vi "PCU_Get_Device_ID.vi"(8 "error in (no error)":errorcluster, 11 ".NET Reference in":refnum<k24>) -> (0 "error out":errorcluster, 2 "id":string[](array[string]), 3 "Reference out":refnum<k24>)   [LabVIEW 2017]
uses:
  D:/test/FULLband-sts/Fullband_Sample/DLL/InstrumentDLL.dll
  DLL/InstrumentDLL.dll
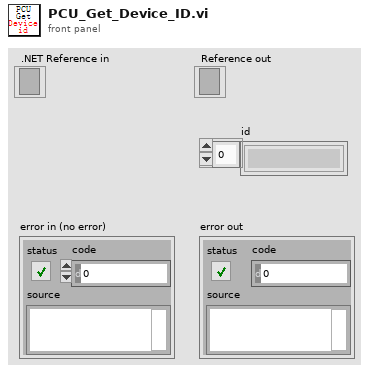
[diagram p1: front panel]
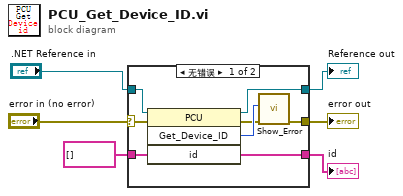
[diagram p0: block diagram]
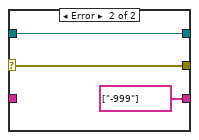
[diagram p2: hidden frame]
diagram:
  n1 = case shown="无错误" "error in (no error)" {
    selector: "error in (no error)" -> [w7 w17]
    tunnel: [w14 string[] ["-999"] ("id")] -> w6
    tunnel: string[] [] ("id") -> [w13 _]
    tunnel: ".NET Reference in" -> [w12 w16]
    tunnel: [w11 w16] -> w3
    tunnel: [w8 w17] -> w2
    frame No Error {
      n2 = invoke on="调用节点" class="PCU" method="Get_Device_ID"(reference=w12, error in=w7, "id"=w13) -> (reference out=w11:refnum<k24>, error out=w9:errorcluster, "Get_Device_ID"=w10:i32, "id"=w14:string[])  [unwired: 1 in]
      n3 = call "Show_Error.vi"("error in (no error)"=w9, "Error"=w10) -> ("error out"=w8:errorcluster)  [unwired: 9 in]
    }
    frame Error {
    }
  }
  "id" <- w6
  "Reference out" <- w3
  "error out" <- w2
